vi "Config Reference Mode.vi"(8 "error in":errorcluster, 9 "Loss Mode (off)":bool, 10 "Capacitance Mode (off)":bool, 11 "VISA resource name":refnum<visa-resource-name>) -> (0 "error out":errorcluster, 3 "VISA resource name out":refnum<visa-resource-name>)   [LabVIEW 2016, in "Andeen-Hagerling 2550.lvlib"]
doc: "This VI changes bridge mode between \"Absolute result mode\" and \"Reference result mode\"."
uses:
  Andeen-Hagerling 2550.lvlib
panel:
  # "Reference Parameters"
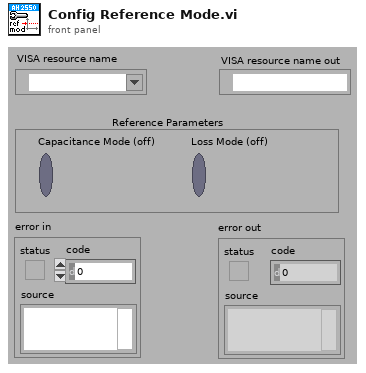
[diagram p1: front panel]
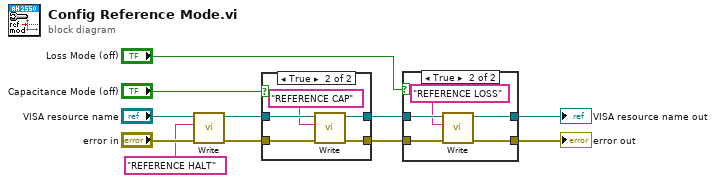
[diagram p0: block diagram]
diagram:
  n1 = call "Write.vi"("error in"="error in", "command"="REFERENCE HALT", "VISA resource name"="VISA resource name") -> ("error out"=w5:errorcluster, "VISA resource name out"=w6:refnum<visa-resource-name>)  [unwired: 7 in]
  n2 = case shown="True" "Capacitance Mode (off)" {
    tunnel: w6 -> [w13 w18]
    tunnel: w5 -> [w12 w17]
    tunnel: [w12 w16] -> w4
    tunnel: [w13 w15] -> w3
    frame False {
    }
    frame True {
      n3 = call "Write.vi"("error in"=w17, "command"="REFERENCE CAP" ("format string"), "VISA resource name"=w18) -> ("error out"=w16:errorcluster, "VISA resource name out"=w15:refnum<visa-resource-name>)  [unwired: 7 in]
    }
  }
  n4 = case shown="True" "Loss Mode (off)" {
    tunnel: [w20 w25] -> w11
    tunnel: [w19 w24] -> w10
    tunnel: w4 -> [w19 w23]
    tunnel: w3 -> [w20 w22]
    frame False {
    }
    frame True {
      n5 = call "Write.vi"("error in"=w23, "command"="REFERENCE LOSS" ("format string"), "VISA resource name"=w22) -> ("error out"=w24:errorcluster, "VISA resource name out"=w25:refnum<visa-resource-name>)  [unwired: 7 in]
    }
  }
  "VISA resource name out" <- w11
  "error out" <- w10
